vi "ProdaNG.ProcessResult.Set.vi"(8 "error in (no error)":errorcluster, 10 "ProcessResult":T1, 11 "dbHandle":i32) -> (0 "error out":errorcluster, 3 "dbHandle":i32)   [LabVIEW 2016]
doc: "This function changes the Process Result that is defined by a ProcessResult structure. A process result can either be set intentionally or leave the check of the process step results and the resulting changes to the DLL. In case, that the DLL changes the Process Result, the mdTime of the according Product is set to the current time.\nThe automatic check stands to the following rules:\n1. It is checked, that the individual Flag in the product is set to 0.\n2. It is checked, if the last process step has already been performed.\nOnly if these two tests are successful, the statusId is set in the process result and only then a further test takes place, to find the status to be set:\n3. It is checked, if all recently performed process steps are finished and have a status of 1 (IO) or 5 (Repeat IO).\nIf the result of the third test is IO, the status 1 is set in the process result, otherwise the status 2 (in Process).\n\nParameter:\nhandle is an Integer, which is returned by the function Login() at the creation of a new connection.\nprocessResult is a pointer on a ProcessResult structure, which elements must be prefilled. The structure must be defined and filled in the calling program. Changes can only be done on the elements statusId, startTime and endTime. If the Endtime is not set, it is automatically filled with the current time by the DLL. \nThe element statusId is of particular importance:\nIf this element is passed with the value -1, the DLL makes a check on the process step results and sets the changeable elements automatically. Otherwise the returned values for status, start time and end time are set. \n\nReturncodes:\n0 No error\n< 0 ORACLE Error code\n6 (ERROR_INVALID_HANDLE) in case of an invalid handle\n1403 Record does not exist"
uses:
  Controls/ProdaNG.ProcessResult.ctl
  Controls/ProdaNG.ProcessResultSize.ctl
  prodllNG.dll
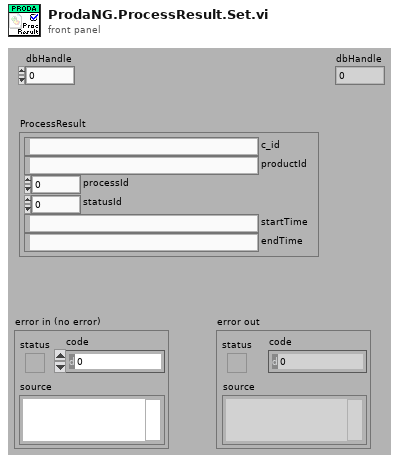
[diagram p1: front panel]
types:
  T1 = typedef "ProdaNG.ProcessResult.ctl" = cluster{"c_id":string, "productId":string, "processId":i32, "statusId":i32, "startTime":string, "endTime":string}
  T2 = typedef "ProdaNG.ProcessResultSize.ctl" = cluster{"c_id":i32, "productId":i32, "processId":i32, "statusId":i32, "startTime":i32, "endTime":i32}
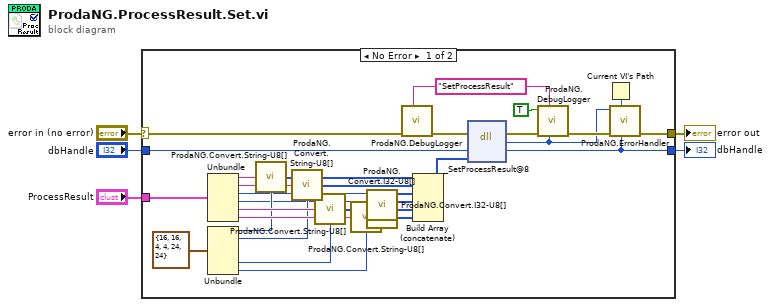
[diagram p0: block diagram]
diagram:
  n1 = case shown="No Error" "error in (no error)" {
    selector: "error in (no error)" -> [w10 w37]
    tunnel: [w7 w37] -> w4
    tunnel: "dbHandle" -> [w9 w36]
    tunnel: [w6 w36] -> w2
    tunnel: "ProcessResult" -> [w8 _]
    frame No Error {
      w30 = "SetProcessResult" ("cmd")
      n2 = Unbundle(w8) -> ("c_id"=w34:string, "productId"=w35:string, "processId"=w20:i32, "statusId"=w19:i32, "startTime"=w32:string, "endTime"=w33:string)
      n3 = Unbundle(T2 {"c_id"=16, "productId"=16, "processId"=4, "statusId"=4, "startTime"=24, "endTime"=24} ("ProcessResultSize")) -> ("c_id"=w24:i32, "productId"=w22:i32, "startTime"=w13:i32, "endTime"=w14:i32)  [unwired: 2 out]
      n4 = call "ProdaNG.Convert.String-U8[].vi"("Input String"=w34, "Size"=w24) -> ("Output"=w23:u8[])
      n5 = call "ProdaNG.Convert.String-U8[].vi"("Input String"=w35, "Size"=w22) -> ("Output"=w21:u8[])
      n6 = call "ProdaNG.Convert.String-U8[].vi"("Input String"=w32, "Size"=w13) -> ("Output"=w15:u8[])
      n7 = call "ProdaNG.Convert.String-U8[].vi"("Input String"=w33, "Size"=w14) -> ("Output"=w16:u8[])
      n8 = call "ProdaNG.Convert.I32-U8[].vi"("32bit integer"=w20) -> ("unsigned byte array"=w18:u8[])  [unwired: 10 in]
      n9 = call "ProdaNG.Convert.I32-U8[].vi"("32bit integer"=w19) -> ("unsigned byte array"=w17:u8[])  [unwired: 10 in]
      n10 = call "ProdaNG.DebugLogger.vi"("cmd"=w30, "error in (no error)"=w10) -> ("error out"=w25:errorcluster)  [unwired: 9 in]
      n11 = Build Array (concatenate)(w23, w21, w18, w17, w15, w16) -> (w11:u8[])
      n12 = dll-call lib="D:/svn/LineTraceSystem/SOFTWARE/sources/Database/ProdaNG/prodllNG.dll" fn="_SetProcessResult@8" ("ProDll.dll:InitProDll")(error in=w25, "dbHandle"=w9, "processResult"=w11) -> (error out=w28:errorcluster, "return type"=w26:i32, "dbHandle"=w6:i32)  [unwired: 3 in, 1 out]
      n13 = call "ProdaNG.DebugLogger.vi"("return type"=w26, "cmd"=w30, "error in (no error)"=w28, "done? (F)"=TRUE) -> ("error out"=w27:errorcluster)  [unwired: 7 in]
      n14 = Current VI's Path() -> (path=w31:path)
      n15 = call "ProdaNG.ErrorHandler.vi"("dbHandleIn"=w6, "Path"=w31, "error in"=w27, "output_parameter"=w26) -> ("error out"=w7:errorcluster)  [unwired: 7 in]
    }
    frame Error {
    }
  }
  "error out" <- w4
  "dbHandle" <- w2
